vi "Commit Device Properties.vi"(0 "Session Handle in":T1, 11 "error in (no error)":errorcluster) -> (4 "Session Handle out":T1, 15 "error out":errorcluster)   [LabVIEW 2015, in "SLSC Switch.lvlib" / "SLSC Session.lvclass"]
uses:
  SLSC Session.lvclass
  Typedefs/Session Handle.ctl
  SLSC Session.lvclass/SLSC Session.ctl
  <vilib>/SLSC/Commit Properties for Devices.vi
  <vilib>/SLSC/SLSC.lvlib
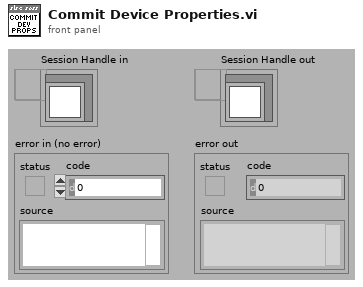
[diagram p1: front panel]
types:
  T1 = typedef "SLSC Switch.lvlib/SLSC Session.lvclass/Session Handle.ctl" = refnum<data-value>
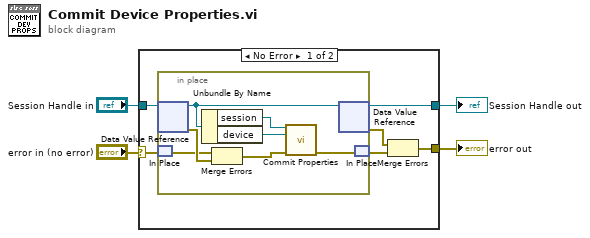
[diagram p0: block diagram]
diagram:
  n1 = case shown="No Error" "error in (no error)" {
    selector: "error in (no error)" -> [w5 w18]
    tunnel: "Session Handle in" -> [w10 w19]
    tunnel: [w9 w19] -> w3
    tunnel: [w6 w18] -> w2
    frame No Error {
      n2 = in-place {
        n3 = in-place-dvr #1(w10) -> (w15:refnum<class "SLSC Session.lvclass">, w17:errorcluster)
        n4 = in-place-match #2(w5) -> (w16:errorcluster)
        n5 = Unbundle By Name(w15) -> ("session"=w14:refnum<k21>, "device"=w13:refnum<k21>)
        n6 = Merge Errors(w16, w17) -> (w12:errorcluster)
        n7 = call-poly <vilib>:"Commit Properties.vi"("session in"=w14, "devices"=w13, "error in (no error)"=w12) -> ("error out"=w11:errorcluster)  [unwired: 11 in, 1 out]
        n8 = in-place-dvr #1(w15) -> (w9:T1, w7:errorcluster)
        n9 = in-place-match #2(w11) -> (w8:errorcluster)
      }
      n10 = Merge Errors(w7, w8) -> (w6:errorcluster)
    }
    frame Error {
    }
  }
  "Session Handle out" <- w3
  "error out" <- w2
